vi "Stop Measurement.vi"(8 "error in":errorcluster, 11 "call id":T1) -> (0 "error out":errorcluster)   [LabVIEW 2025, in "Automotive-Ethernet_LabVIEW.lvlib"]
doc: "Stop the measurement."
uses:
  Automotive-Ethernet_LabVIEW.lvlib
  <vilib>/gRPC/LabVIEW gRPC Library/Shared/grpcId.ctl
  <vilib>/gRPC/Generated APIs/ni/measurementlink/measurement/v2/Measurement Service Client V2/Measurement Service Client V2.lvlib
  <vilib>/gRPC/LabVIEW gRPC Library/grpc-lvsupport-release.lvlib
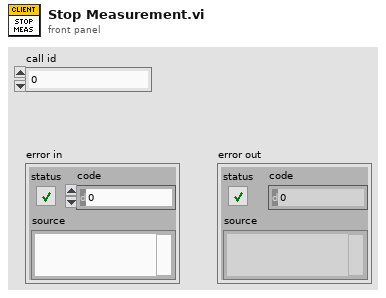
[diagram p1: front panel]
types:
  T1 = typedef "grpc-lvsupport-release.lvlib/grpcId.ctl" = u64
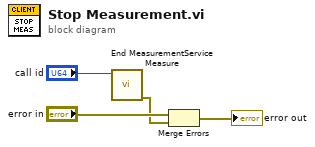
[diagram p0: block diagram]
diagram:
  n1 = call <vilib>:"End MeasurementService Measure.vi"("Call ID in"="call id") -> ("error out"=w1:errorcluster)  [unwired: 9 in, 1 out]
  n2 = Merge Errors("error in", w1) -> (→"error out":errorcluster)
